vi "Register Sessions.vi"(8 "error in":errorcluster, 11 "session reservation in":refnum<class "Session Reservation.lvclass">) -> (0 "error out":errorcluster, 3 "session reservation out":refnum<class "Session Reservation.lvclass">)   [LabVIEW 2020, in "MeasurementLink Session Management.lvlib" / "Session Reservation.lvclass"]
doc: "Registers sessions with the session management service for shared use."
uses:
  Session Reservation.lvclass
  Session Reservation.lvclass/Session Reservation.ctl
  MeasurementLink Session Management Client/RPC Messages/ni_measurementlink_sessionmanagement_v1_RegisterSessionsRequest.ctl
  MeasurementLink Session Management Client/RPC Messages/ni_measurementlink_sessionmanagement_v1_SessionInformation.ctl
  MeasurementLink Session Management Client/RPC Messages/nidevice_grpc_Session.ctl
  MeasurementLink Session Management Client/RPC Messages/ni_measurementlink_sessionmanagement_v1_ChannelMapping.ctl
  MeasurementLink Measurement Server/Helpers/Error Strings Global Internal.vi
  MeasurementLink Session Management Client/MeasurementLink Session Management Client.lvlib
  MeasurementLink Session Management Client Wrapper/MeasurementLink Session Management Client Wrapper.lvlib
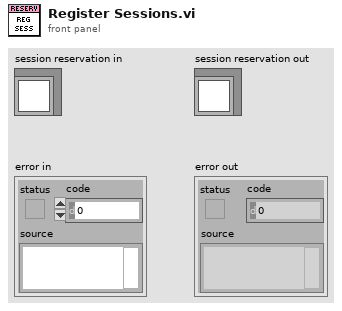
[diagram p1: front panel]
types:
  T1 = typedef "MeasurementLink Session Management Client.lvlib/ni_measurementlink_sessionmanagement_v1_RegisterSessionsRequest.ctl" = cluster{"sessions":T2[]}
  T2 = typedef "MeasurementLink Session Management Client.lvlib/ni_measurementlink_sessionmanagement_v1_SessionInformation.ctl" = cluster{"session":T3, "resource_name":string, "channel_list":string, "instrument_type_id":string, "session_exists":bool, "channel_mappings":T4[]}
  T3 = typedef "MeasurementLink Session Management Client.lvlib/nidevice_grpc_Session.ctl" = cluster{"name":string}
  T4 = typedef "MeasurementLink Session Management Client.lvlib/ni_measurementlink_sessionmanagement_v1_ChannelMapping.ctl" = cluster{"pin_or_relay_name":string, "site":i32, "channel":string}
  T5 = typedef "MeasurementLink Session Management.lvlib/Session Reservation.lvclass/Data.ctl" = cluster{"session and driver infos":T6[], "pin or relay names":string[], "connection map":refnum<class "Connection Map.lvclass">, "pin map context":T8, "reservation observer":refnum<class "IReservationObserver.lvclass">, "dvr valid":bool}
  T6 = typedef "MeasurementLink Session Management.lvlib/Session Reservation.lvclass/Session and Driver Info.ctl" = cluster{"session info":T2, "session":variant, "instrument":refnum<class "IInstrument.lvclass">, "initialize and close session behavior":T7}
  T7 = typedef "MeasurementLink Instrument.lvlib/IInstrument.lvclass/Initialize and Close Session Behavior.ctl" = enum16{"Initialize and Close", "Attach and Detach", "Initialize and Detach", "Attach and Close"}
  T8 = typedef "MeasurementLink Session Management Client.lvlib/ni_measurementlink_PinMapContext.ctl" = cluster{"pin_map_id":string, "sites":i32[]}
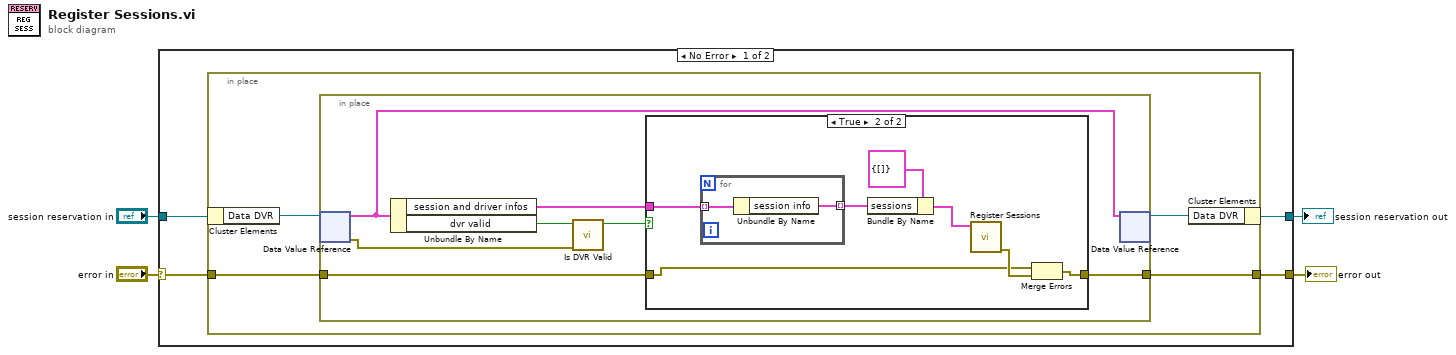
[diagram p0: block diagram]
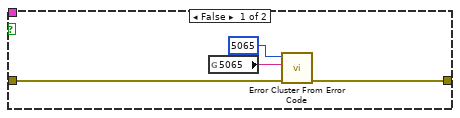
[diagram p2: hidden frame]
diagram:
  n1 = case shown="No Error" "error in" {
    selector: "error in" -> [w6 w33]
    tunnel: [w7 w34] -> w2
    tunnel: "session reservation in" -> [w8 w34]
    tunnel: [w5 w33] -> w1
    frame No Error {
      n2 = in-place {
        in-place-border: w6 -> [w10]
        in-place-border: [w9] -> w5
        n3 = in-place-cluster #1(w8) -> ("Data DVR"=w12:refnum<data-value>)
        n4 = in-place {
          in-place-border: w10 -> [w15]
          in-place-border: [w14] -> w9
          n5 = in-place-dvr #2(w12) -> (w13:T5, w18:errorcluster)
          n6 = Unbundle By Name(w13) -> ("session and driver infos"=w16:T6[], "dvr valid"=w19:bool)
          n7 = call "Is DVR Valid.vi"("dvr error in"=w18, "dvr valid"=w19) -> ("dvr valid"=w17:bool)  [unwired: 9 in]
          n8 = case shown="True" w17 {
            tunnel: w16 -> [_ w27]
            tunnel: w15 -> [w22 w25]
            tunnel: [w21 w24] -> w14
            frame False {
              n9 = global read "Error Strings Global Internal.vi" "5065"() -> (w23:string)
              n10 = call <vilib>:"Error Cluster From Error Code.vi"("error in (no error)"=w22, "error message (\"\")"=w23, "error code (0)"=5065) -> ("error out"=w21:errorcluster)  [unwired: 6 in]
            }
            frame True {
              n11 = for {
                tunnel: w27 -> [w32] mode=indexing
                tunnel: [w31] -> w29 mode=indexing
                n12 = Unbundle By Name(w32) -> ("session info"=w31:T2)
              }
              n13 = Bundle By Name(cluster=T1 {"sessions"=[]} ("Request Data"), "sessions"=w29) -> (w28:T1)
              n14 = call "Register Sessions.vi"("request data"=w28) -> ("error out"=w26:errorcluster)  [unwired: 9 in, 1 out]
              n15 = Merge Errors(w25, w26) -> (w24:errorcluster)
            }
          }
          n16 = in-place-dvr #2(w13) -> (w11:refnum<data-value>)  [unwired: 1 out]
        }
        n17 = in-place-cluster #1("Data DVR"=w11) -> (w7:refnum<class "Session Reservation.lvclass">)
      }
    }
    frame Error {
    }
  }
  "error out" <- w1
  "session reservation out" <- w2
